vi "iTC_Readout.vi"() -> ()   [LabVIEW 2009]
panel:
  out "millisecond timer value":u32
  out "CCS Resistance":dynamicdata(graph)
  out "CCS Temperature":dbl(slide) scale=0.0..100.0
  in  "Samples Per Second 6":dbl=15.0
  out "CCS Temperature":string
  out "CCS Resistance":dbl(knob) scale=0.0..500.0
  out "CCS Resistance":string
  out "CCS Temperature":dynamicdata(graph)
  in  "Samples Per Second 5":dbl=15.0
  out "Allen Bradley Temperature":dbl(slide) scale=0.0..500.0
  out "Allen Bradley Temperature":string
  out "Allen Bradley Temperature":dynamicdata(graph)
  in  "Samples Per Second 4":dbl=15.0
  out "Allen Bradley Resistance":dbl(knob) scale=0.3..300.0
  out "Allen Bradley Resistance":string
  out "Allen Bradley Resistance":dynamicdata(graph)
  in  "Samples Per Second 3":dbl=15.0
  in  "Samples Per Second 2":dbl=15.0
  in  "Samples Per Second":dbl=15.0
  in  "stop 2":bool
  out "Heartbeat":bool
  out "Cernox Temp":string
  out "Cernox Temperature":dynamicdata(graph)
  out "Cernox Temp":dbl(slide) scale=0.0..320.0
  out "Cernox Resistance":dynamicdata(graph)
  out "Cernox Resistance":dbl(knob) scale=0.0..300.0
  out "Cernox Resistance":string
  in  "stop":bool
  out "Measurement":bool caption="Taken"
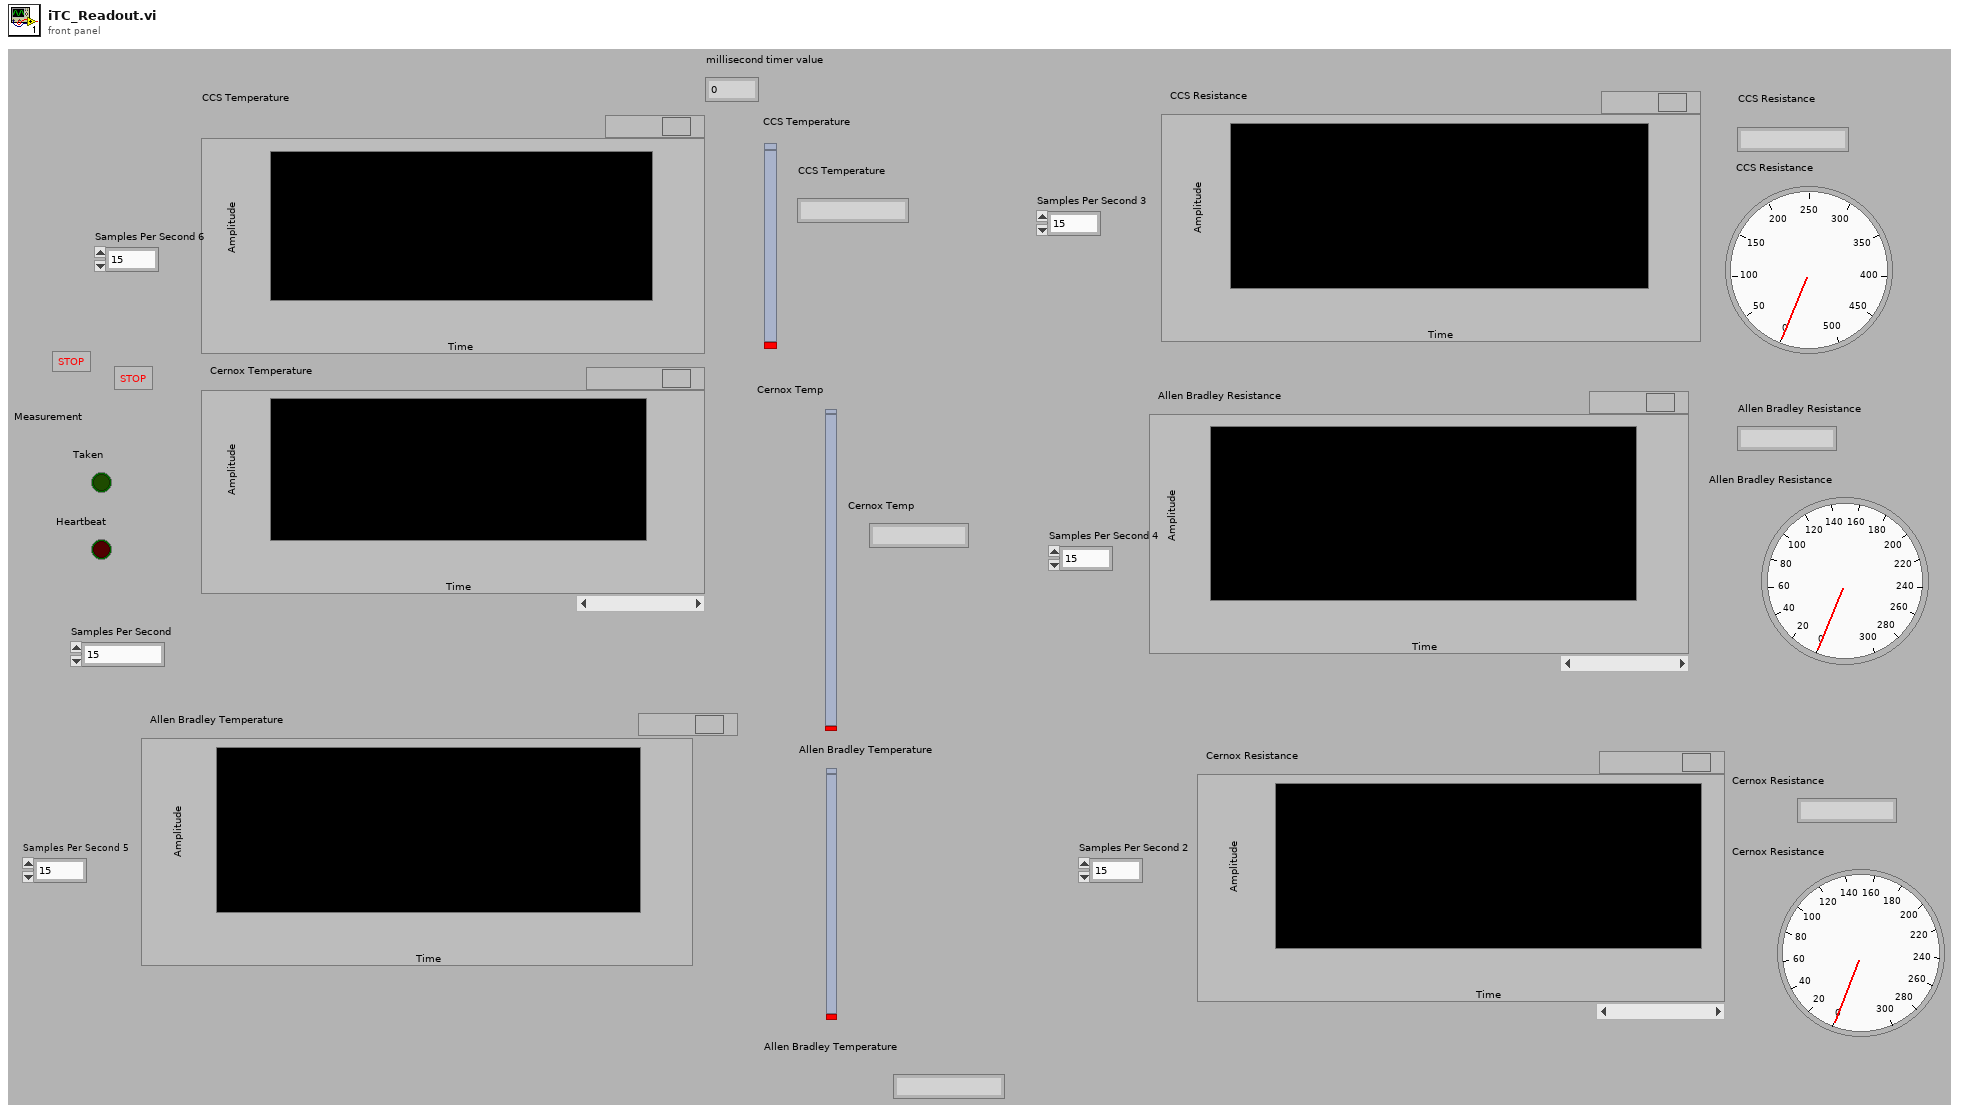
[diagram p1: front panel]
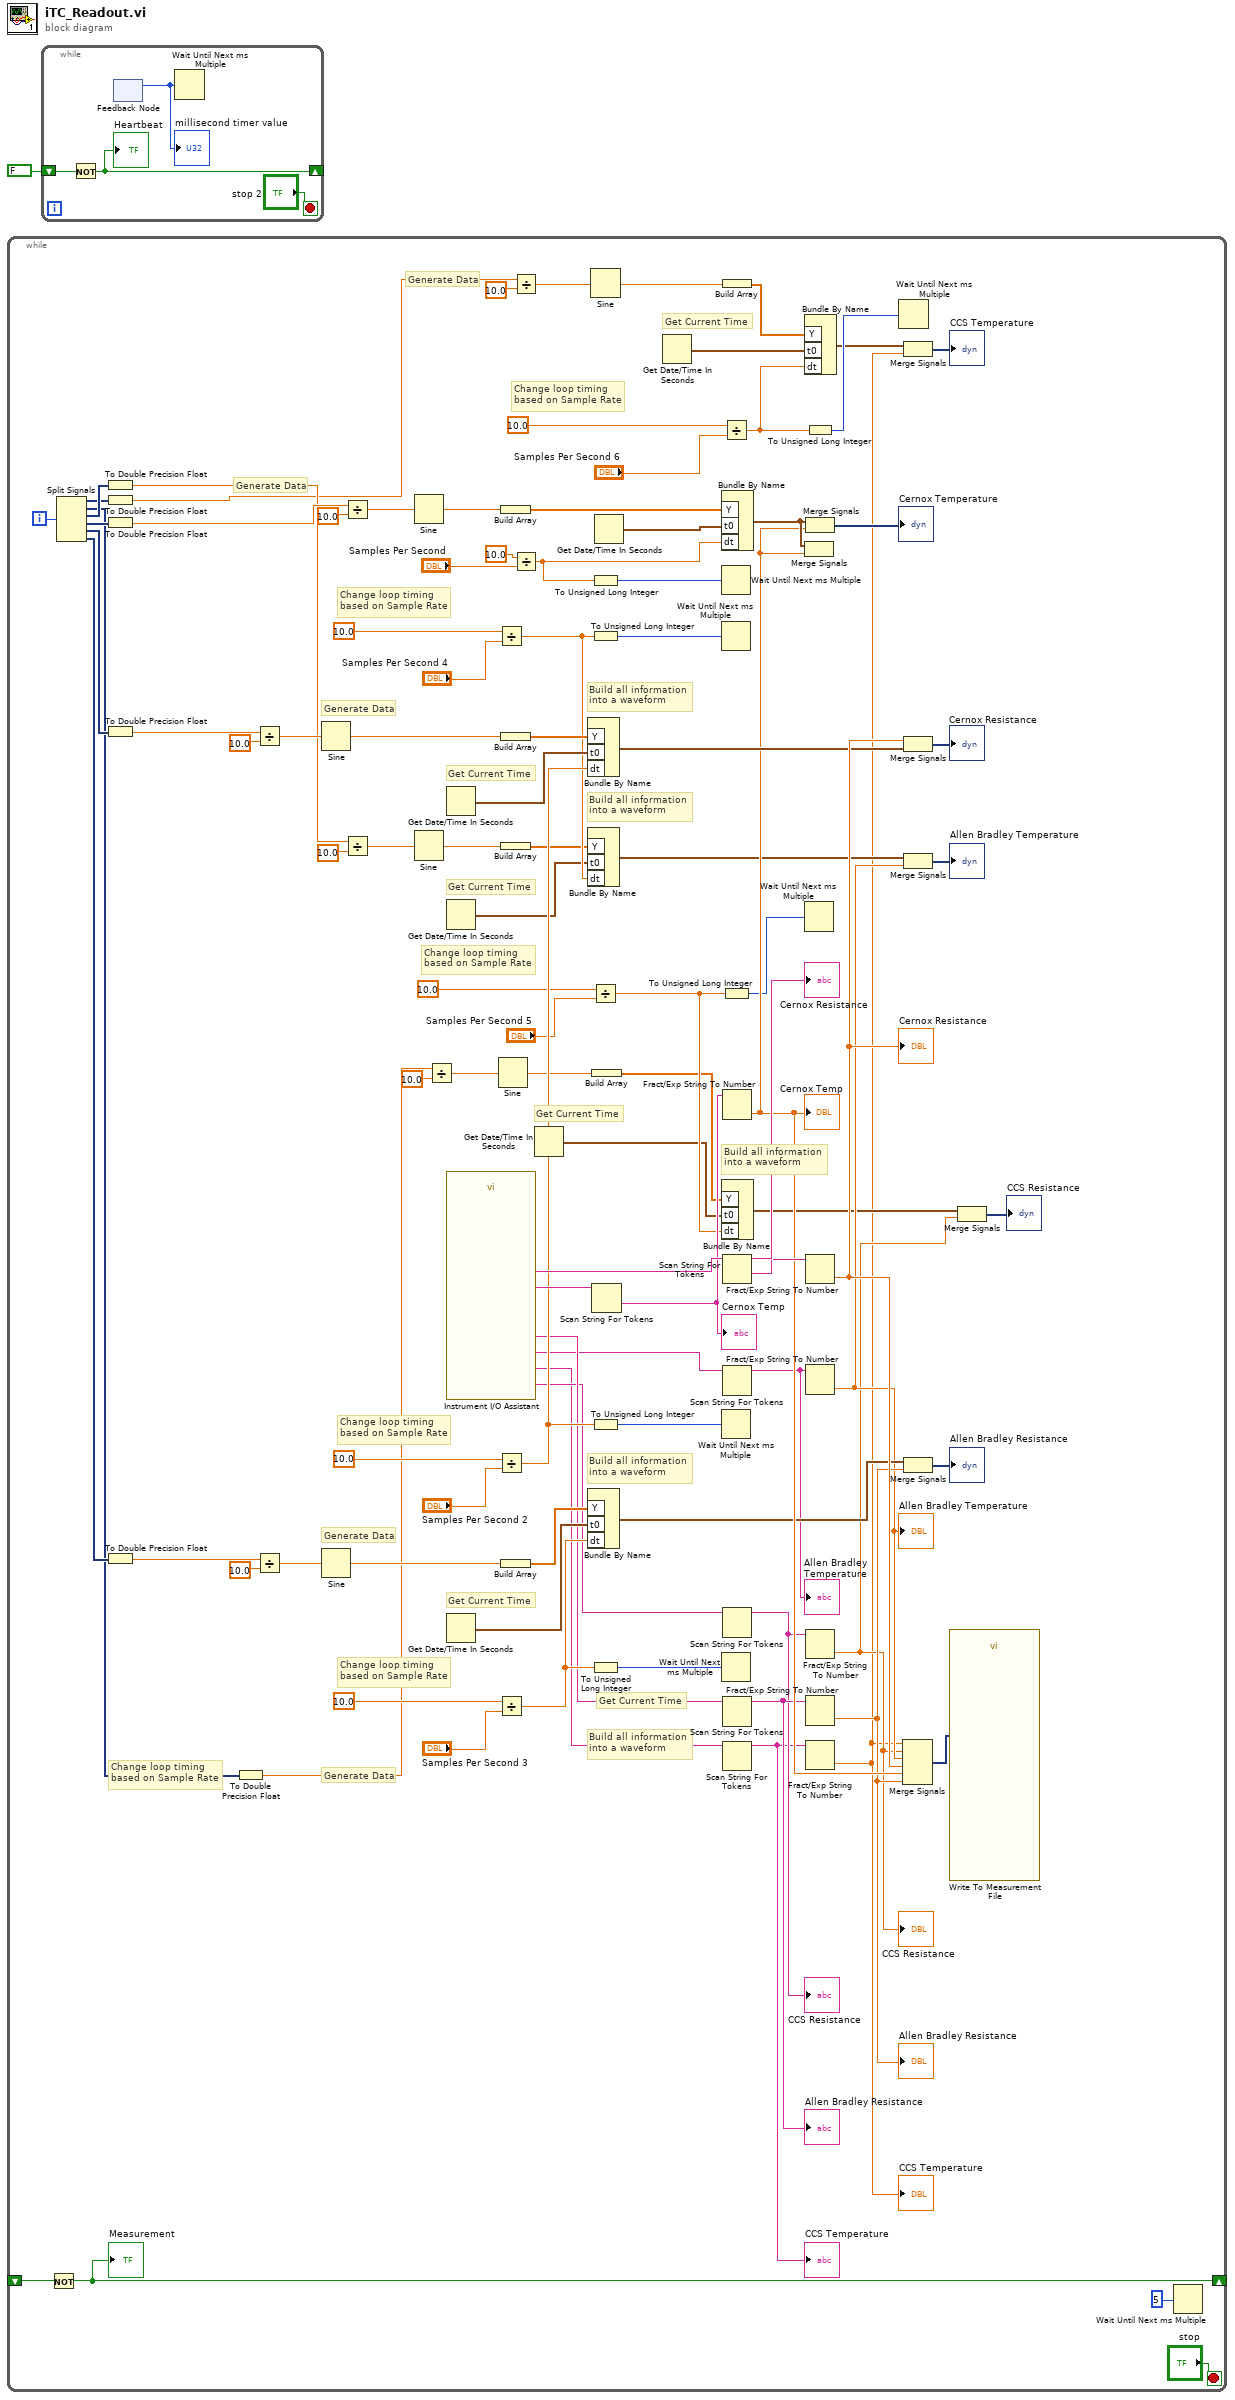
[diagram p0: block diagram]
diagram:
  n1 = while {
    shift-right: [w103] -> _
    shift-left: _ -> [w104]
    i -> [w72]
    stop <- "stop" stop-if-true
    # "Build all information\ninto a waveform"
    # "Change loop timing\nbased on Sample Rate"
    # "Get Current Time"
    # "Generate Data"
    # "Build all information\ninto a waveform"
    # "Change loop timing\nbased on Sample Rate"
    # "Get Current Time"
    # "Generate Data"
    # "Build all information\ninto a waveform"
    # "Change loop timing\nbased on Sample Rate"
    # "Get Current Time"
    # "Generate Data"
    # "Build all information\ninto a waveform"
    # "Change loop timing\nbased on Sample Rate"
    # "Get Current Time"
    # "Generate Data"
    # "Build all information\ninto a waveform"
    # "Change loop timing\nbased on Sample Rate"
    # "Get Current Time"
    # "Generate Data"
    # "Change loop timing\nbased on Sample Rate"
    # "Get Current Time"
    n2 = Not(x=w104) -> (.not. x?=w103:bool)
    "Measurement" <- w103
    n3 = Split Signals(w72) -> (w6:dynamicdata, w22:dynamicdata, w37:dynamicdata, w71:dynamicdata, w70:dynamicdata, w57:dynamicdata)  [unwired: 6 in]
    n4 = To Double Precision Float(number=w37) -> (double precision float=w45:dbl)
    n5 = To Double Precision Float(number=w6) -> (double precision float=w12:dbl)
    n6 = To Double Precision Float(number=w71) -> (double precision float=w91:dbl)
    n7 = To Double Precision Float(number=w70) -> (double precision float=w78:dbl)
    n8 = To Double Precision Float(number=w57) -> (double precision float=w61:dbl)
    n9 = To Double Precision Float(number=w22) -> (double precision float=w29:dbl)
    n10 = Divide(x=w78, y=10.0) -> (x/y=w76:dbl)
    n11 = Divide(x=w61, y=10.0) -> (x/y=w58:dbl)
    n12 = Sine(x=w76) -> (sin(x)=w81:dbl)
    n13 = Sine(x=w58) -> (sin(x)=w64:dbl)
    n14 = Divide(x=w91, y=10.0) -> (x/y=w94:dbl)
    n15 = Divide(x=w45, y=10.0) -> (x/y=w42:dbl)
    n16 = Sine(x=w94) -> (sin(x)=w88:dbl)
    n17 = Sine(x=w42) -> (sin(x)=w48:dbl)
    n18 = Divide(x=w29, y=10.0) -> (x/y=w26:dbl)
    n19 = Get Date/Time In Seconds() -> (seconds since 1Jan1904=w83:timestamp)
    n20 = Get Date/Time In Seconds() -> (seconds since 1Jan1904=w50:timestamp)
    n21 = call "Instrument I/O Assistant"() -> ("CCS Resistance"=w24:string, "CCS Temperature"=w20:string, "Allen Bradley Temperature"=w39:string, "Allen Bradley Resistance"=w55:string, "Cernox Temp"=w99:string, "Cernox Resistance"=w101:string)  [unwired: 21 in, 1 out]
    n22 = Get Date/Time In Seconds() -> (seconds since 1Jan1904=w66:timestamp)
    n23 = Divide(x=10.0, y="Samples Per Second 4") -> (x/y=w51:dbl)
    n24 = Divide(x=10.0, y="Samples Per Second 2") -> (x/y=w84:dbl)
    n25 = Divide(x=10.0, y="Samples Per Second 3") -> (x/y=w67:dbl)
    n26 = Sine(x=w26) -> (sin(x)=w32:dbl)
    n27 = Build Array(w88) -> (w87:dbl[])
    n28 = Build Array(w81) -> (w82:dbl[])
    n29 = Build Array(w48) -> (w49:dbl[])
    n30 = Build Array(w64) -> (w65:dbl[])
    n31 = Divide(x=w12, y=10.0) -> (x/y=w9:dbl)
    n32 = Divide(x=10.0, y="Samples Per Second") -> (x/y=w85:dbl)
    n33 = Get Date/Time In Seconds() -> (seconds since 1Jan1904=w34:timestamp)
    n34 = Bundle By Name("Y"=w82, "t0"=w83, "dt"=w84) -> (w73:waveform(dbl))  [unwired: 1 in]
    n35 = Bundle By Name("Y"=w49, "t0"=w50, "dt"=w51) -> (w41:waveform(dbl))  [unwired: 1 in]
    n36 = Bundle By Name("Y"=w65, "t0"=w66, "dt"=w67) -> (w56:waveform(dbl))  [unwired: 1 in]
    n37 = Sine(x=w9) -> (sin(x)=w15:dbl)
    n38 = To Unsigned Long Integer(number=w85) -> (unsigned 32bit integer=w92:u32)
    n39 = To Unsigned Long Integer(number=w51) -> (unsigned 32bit integer=w44:u32)
    n40 = Divide(x=10.0, y="Samples Per Second 5") -> (x/y=w35:dbl)
    n41 = To Unsigned Long Integer(number=w84) -> (unsigned 32bit integer=w77:u32)
    n42 = To Unsigned Long Integer(number=w67) -> (unsigned 32bit integer=w60:u32)
    n43 = Build Array(w32) -> (w33:dbl[])
    n44 = Scan String For Tokens(9:w99) -> (1:w97:string)  [unwired: 5 in, 3 out]
    "Cernox Temp" <- w97
    n45 = Get Date/Time In Seconds() -> (seconds since 1Jan1904=w86:timestamp)
    n46 = Get Date/Time In Seconds() -> (seconds since 1Jan1904=w17:timestamp)
    n47 = Bundle By Name("Y"=w87, "t0"=w86, "dt"=w85) -> (w69:waveform(dbl))  [unwired: 1 in]
    n48 = Wait Until Next ms Multiple(millisecond multiple=w92) -> ()  [unwired: 1 out]
    n49 = Wait Until Next ms Multiple(millisecond multiple=w44) -> ()  [unwired: 1 out]
    n50 = Bundle By Name("Y"=w33, "t0"=w34, "dt"=w35) -> (w25:waveform(dbl))  [unwired: 1 in]
    n51 = Wait Until Next ms Multiple(millisecond multiple=w77) -> ()  [unwired: 1 out]
    n52 = Wait Until Next ms Multiple(millisecond multiple=w60) -> ()  [unwired: 1 out]
    n53 = Build Array(w15) -> (w16:dbl[])
    n54 = Divide(x=10.0, y="Samples Per Second 6") -> (x/y=w18:dbl)
    n55 = To Unsigned Long Integer(number=w35) -> (unsigned 32bit integer=w28:u32)
    n56 = Fract/Exp String To Number(string=w97) -> (number=w68:dbl)  [unwired: 3 in, 1 out]
    "Cernox Temp" <- w68
    n57 = Scan String For Tokens(9:w101) -> (1:w100:string, 3:→"Cernox Resistance":string)  [unwired: 5 in, 2 out]
    n58 = Scan String For Tokens(9:w39) -> (3:w38:string)  [unwired: 5 in, 3 out]
    "Allen Bradley Temperature" <- w38
    n59 = Scan String For Tokens(9:w24) -> (3:w23:string)  [unwired: 5 in, 3 out]
    "CCS Resistance" <- w23
    n60 = Scan String For Tokens(9:w55) -> (3:w53:string)  [unwired: 5 in, 3 out]
    "Allen Bradley Resistance" <- w53
    n61 = Scan String For Tokens(9:w20) -> (3:w19:string)  [unwired: 5 in, 3 out]
    "CCS Temperature" <- w19
    n62 = Bundle By Name("Y"=w16, "t0"=w17, "dt"=w18) -> (w8:waveform(dbl))  [unwired: 1 in]
    n63 = Merge Signals(w69, w68) -> ()  [unwired: 1 out]
    n64 = Wait Until Next ms Multiple(millisecond multiple=w28) -> ()  [unwired: 1 out]
    n65 = To Unsigned Long Integer(number=w18) -> (unsigned 32bit integer=w11:u32)
    n66 = Merge Signals(w69, w68) -> (→"Cernox Temperature":dynamicdata)
    n67 = Fract/Exp String To Number(string=w100) -> (number=w75:dbl)  [unwired: 3 in, 1 out]
    "Cernox Resistance" <- w75
    n68 = Fract/Exp String To Number(string=w38) -> (number=w36:dbl)  [unwired: 3 in, 1 out]
    "Allen Bradley Temperature" <- w36
    n69 = Fract/Exp String To Number(string=w23) -> (number=w21:dbl)  [unwired: 3 in, 1 out]
    "CCS Resistance" <- w21
    n70 = Fract/Exp String To Number(string=w53) -> (number=w52:dbl)  [unwired: 3 in, 1 out]
    "Allen Bradley Resistance" <- w52
    n71 = Fract/Exp String To Number(string=w19) -> (number=w5:dbl)  [unwired: 3 in, 1 out]
    "CCS Temperature" <- w5
    n72 = Wait Until Next ms Multiple(millisecond multiple=w11) -> ()  [unwired: 1 out]
    n73 = Merge Signals(w5, w21, w36, w75, w68, w52) -> (w98:dynamicdata)
    n74 = Merge Signals(w8, w5) -> (→"CCS Temperature":dynamicdata)
    n75 = Merge Signals(w75, w73) -> (→"Cernox Resistance":dynamicdata)
    n76 = Merge Signals(w41, w36) -> (→"Allen Bradley Temperature":dynamicdata)
    n77 = Merge Signals(w56, w52) -> (→"Allen Bradley Resistance":dynamicdata)
    n78 = call "Write To Measurement File"("Signals"=w98) -> ()  [unwired: 16 in, 3 out]
    n79 = Merge Signals(w25, w21) -> (→"CCS Resistance":dynamicdata)
    n80 = Wait Until Next ms Multiple(millisecond multiple=u32 5) -> ()  [unwired: 1 out]
  }
  n81 = while {
    shift-right: [w108] -> _
    shift-left: FALSE -> [w109]
    stop <- "stop 2" stop-if-true
    n82 = Not(x=w109) -> (.not. x?=w108:bool)
    "Heartbeat" <- w108
    n83 = feedback #1() -> (w105:u32)  [unwired: 1 in]
    "millisecond timer value" <- w105
    n84 = Wait Until Next ms Multiple(millisecond multiple=w105) -> (millisecond timer value=w106:u32)
  }
